vi "Send single trigger.vi"(8 "error in (no error)":errorcluster, 11 "SA-FSW in":refnum<class "SA-FSW.lvclass">) -> (0 "error out":errorcluster, 3 "SA-FSW out":refnum<class "SA-FSW.lvclass">)   [LabVIEW 2020, in "SA-FSW.lvclass"]
uses:
  SA-FSW.lvclass
  C:/Sandbox/Git_Sandbox/WiSpry Test Framework source code (LV20)/WiSpry Test Framework/Instruments/Instrument.lvclass
  C:/Sandbox/Git_Sandbox/WiSpry Test Framework source code (LV20)/WiSpry Test Framework/Instruments/Spectrum Analyzer/Spectrum Analyzer.lvclass
  Spectrum Analyzer.lvclass/Spectrum Analyzer.ctl
  Instrument.lvclass/Instrument.ctl
  Instrument.lvclass
  Spectrum Analyzer.lvclass
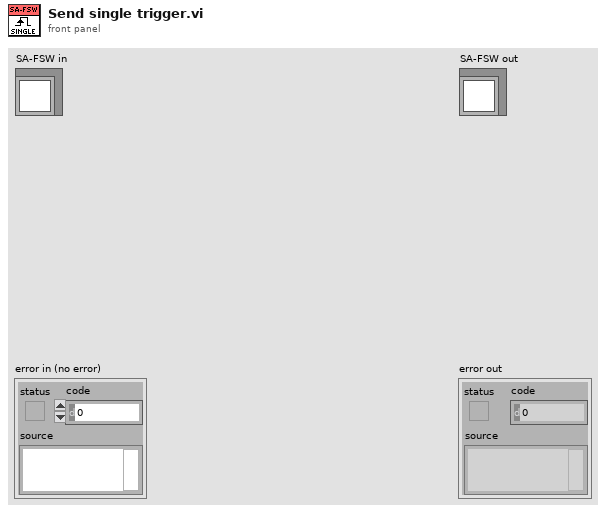
[diagram p1: front panel]
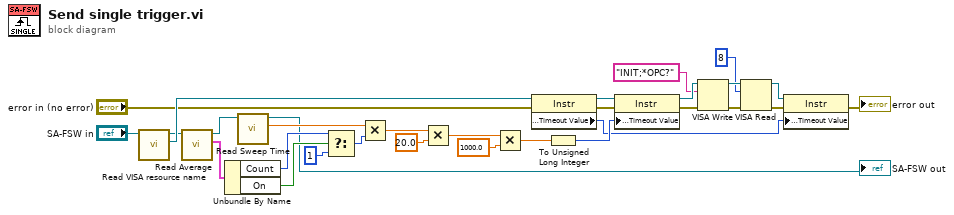
[diagram p0: block diagram]
diagram:
  n1 = call "Read VISA resource name.vi"("Instrument in"="SA-FSW in") -> ("VISA resource name"=w29:refnum<visa-resource-name>, "Instrument out"=w27:refnum<class "SA-FSW.lvclass">)  [unwired: 9 in]
  n2 = call "Read Average.vi"("Spectrum Analyzer in"=w27) -> ("Average"=w25:cluster{"Count":u32, "On":bool}, "Spectrum Analyzer out"=w26:refnum<class "SA-FSW.lvclass">)  [unwired: 9 in]
  n3 = Unbundle By Name(w25) -> ("Count"=w23:u32, "On"=w24:bool)
  n4 = call "Read Sweep Time.vi"("Spectrum Analyzer in"=w26) -> ("Sweep Time"=w21:dbl, "Spectrum Analyzer out"=→"SA-FSW out":refnum<class "SA-FSW.lvclass">)  [unwired: 9 in]
  n5 = Select(t=w23, s=w24, f=u32 1) -> (s? t:f=w20:u32)
  n6 = Multiply(x=w21, y=w20) -> (x*y=w19:dbl)
  n7 = Multiply(x=w19, y=20.0) -> (x*y=w17:dbl)
  n8 = Multiply(x=w17, y=1000.0) -> (x*y=w13:dbl)
  n9 = property class="Instr"(reference=w29, error in="error in (no error)") -> (reference out=w15:refnum<visa-resource-name>, error out=w14:errorcluster, "General Settings:Timeout Value"=w1:u32)
  n10 = To Unsigned Long Integer(number=w13) -> (unsigned 32bit integer=w12:u32)
  n11 = property class="Instr"(reference=w15, error in=w14, "General Settings:Timeout Value"=w12) -> (reference out=w11:refnum<visa-resource-name>, error out=w10:errorcluster)
  n12 = VISA Write(VISA resource name=w11, write buffer="INIT;*OPC?", error in (no error)=w10) -> (VISA resource name out=w7:refnum<visa-resource-name>, error out=w8:errorcluster)  [unwired: 1 out]
  n13 = VISA Read(VISA resource name=w7, byte count=u32 8, error in (no error)=w8) -> (VISA resource name out=w4:refnum<visa-resource-name>, error out=w3:errorcluster)  [unwired: 2 out]
  n14 = property class="Instr"(reference=w4, error in=w3, "General Settings:Timeout Value"=w1) -> (error out=→"error out":errorcluster)  [unwired: 1 out]
